vi "Insert Into Array (Single).vi"(8 "index":i32, 9 "JSON Value in":refnum<class "JSON Value.lvclass">, 11 "JSON Value in":refnum<class "JSON Value.lvclass">) -> (3 "JSON Value out":refnum<class "JSON Value.lvclass">)   [LabVIEW 2016, in "JSON Value.lvclass"]
doc: "Inserts an element or subarray into a JSON array at the point you specify in index."
uses:
  JSON Value.lvclass
  JSON Value.lvclass/JSON Value.ctl
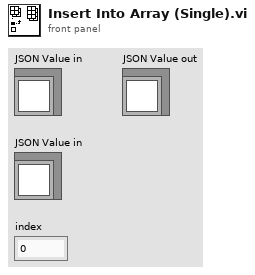
[diagram p1: front panel]
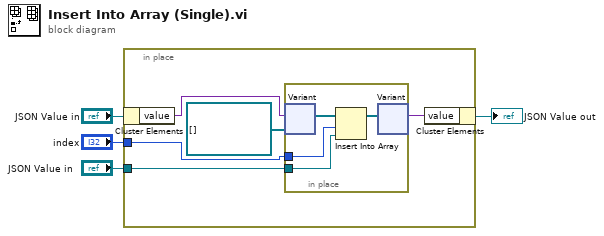
[diagram p0: block diagram]
diagram:
  n1 = in-place {
    in-place-border: "JSON Value in" -> [w8]
    in-place-border: "index" -> [w9]
    n2 = in-place-cluster #1("JSON Value in") -> ("value"=w7:variant)
    n3 = in-place {
      in-place-border: w9 -> [w13]
      in-place-border: w8 -> [w12]
      n4 = in-place-variant #2(w7, refnum<class "JSON Value.lvclass">[] [] ("output array")) -> (w11:refnum<class "JSON Value.lvclass">[])  [unwired: 1 out]
      n5 = Insert Into Array(array=w11, index=w13, new element=w12) -> (w10:refnum<class "JSON Value.lvclass">[])
      n6 = in-place-variant #2(w10) -> (w5:variant)  [unwired: 1 out]
    }
    n7 = in-place-cluster #1("value"=w5) -> (→"JSON Value out":refnum<class "JSON Value.lvclass">)
  }
